vi "BGA244_Main.vi"(7 "stop_external":refnum<vi>, 8 "cluster_ref_BGA244":T1) -> ()   [LabVIEW 2019]
uses:
  cluster_ref_BGA244.ctl
panel:
  in  "Logging":bool=TRUE
  in  "meas_interval":i32=1000 caption="Measurement interval (ms)"
  out "mode":string
  in  "He/Air Mode Button":bool
  out "Purity Meter":dbl(knob) caption="Purity (%)" scale=0.0..100.0 scale format="%#.2f"
  in  "He Mode Button":bool
  in  "O2/N2 Mode Button":bool
  out "gas 2":string
  out "gas 1":string
  out "Purity Chart":waveform(dbl)[](graph)
  out "Status":bool
  in  "VISA":refnum<visa-resource-name>="COM18"
  out "Last measured":timestamp format="%<%Y-%m-%d %H:%M:%S>T"
  in  "Stop":bool
  # "Gas Analyzer Panel"
  # "1333-74-0: H2\n7440-59-7: He\n7727-37-9: N2\n7782-44-7: O2\n7740-37-1: Ar\n132259-10-0: Air"
  # "BGA244"
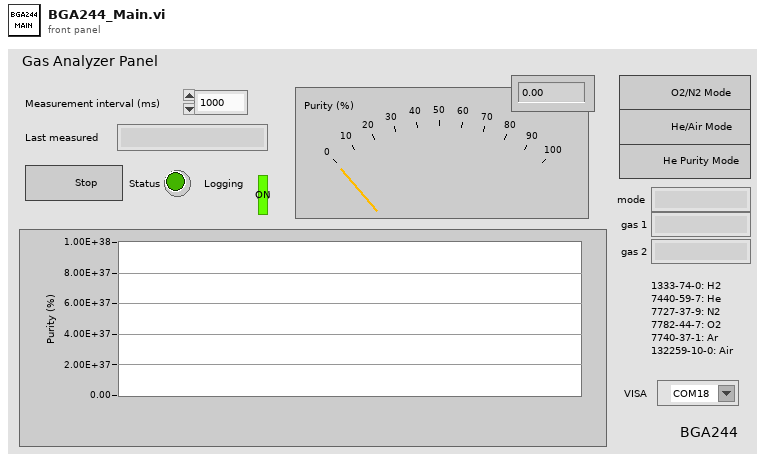
[diagram p1: front panel]
types:
  T1 = typedef "cluster_ref_BGA244.ctl" = cluster{"Status":refnum<vi>, "purity":refnum<vi>}
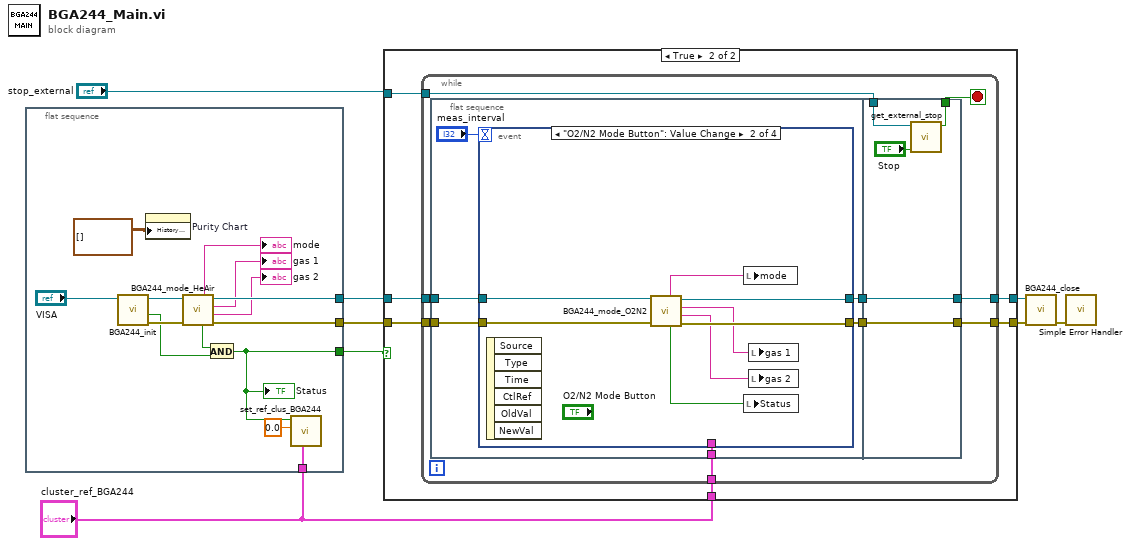
[diagram p0: block diagram]
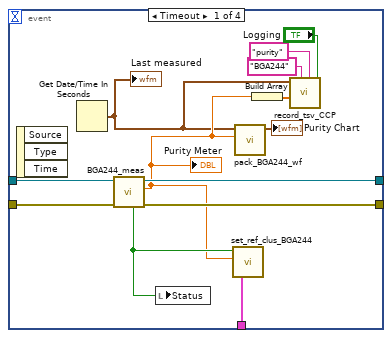
[diagram p3: hidden frame]
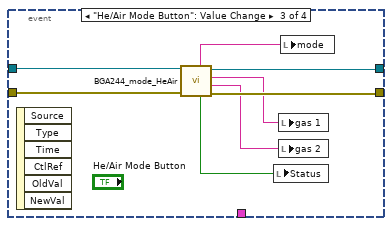
[diagram p4: hidden frame]
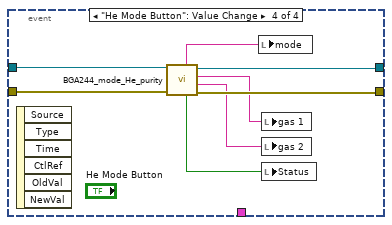
[diagram p5: hidden frame]
diagram:
  n1 = flat-sequence {
    tunnel: [w17] -> w6
    tunnel: [w19] -> w7
    tunnel: "cluster_ref_BGA244" -> [w12]
    tunnel: [w9] -> w1
    frame #0 {
      n2 = call "BGA244_init.vi"("VISA in"="VISA") -> ("error out"=w18:errorcluster, "status"=w14:bool, "VISA out"=w20:refnum<visa-resource-name>)  [unwired: 8 in]
      n3 = property on="Purity Chart" class="WFChart (strict)"("History Data"=waveform(dbl)[][] []) -> ()  [unwired: 2 in, 2 out]
      n4 = call "BGA244_mode_HeAir.vi"("error in"=w18, "VISA in"=w20) -> ("error out"=w17:errorcluster, "gas 2"=→"gas 2":string, "gas 1"=→"gas 1":string, "VISA out"=w19:refnum<visa-resource-name>, "status"=w13:bool, "mode"=→"mode":string)  [unwired: 4 in]
      n5 = And(x=w13, y=w14) -> (x .and. y?=w9:bool)
      "Status" <- w9
      n6 = call "set_ref_clus_BGA244.vi"("cluster_ref_BGA244"=w12, "purity"=0.0, "status"=w9) -> ()  [unwired: 9 in]
    }
  }
  n7 = case shown="True" w1 {
    tunnel: "stop_external" -> [_ w30]
    tunnel: w7 -> [w24 w29]
    tunnel: w6 -> [w23 w28]
    tunnel: [w23 w27] -> w5
    tunnel: [w24 w26] -> w4
    tunnel: "cluster_ref_BGA244" -> [_ w25]
    frame False {
    }
    frame True {
      n8 = while {
        tunnel: w25 -> [w39]
        tunnel: w30 -> [w32]
        tunnel: w29 -> [w38]
        tunnel: w28 -> [w37]
        tunnel: [w36] -> w27
        tunnel: [w35] -> w26
        stop <- w31 stop-if-true
        n9 = flat-sequence {
          tunnel: w39 -> [w45]
          tunnel: w38 -> [w44]
          tunnel: w37 -> [w43]
          tunnel: [w42] -> w34
          tunnel: [w41] -> w33
          tunnel: [w86] -> w35
          tunnel: [w87] -> w36
          tunnel: w34 -> [w87]
          tunnel: w33 -> [w86]
          tunnel: w32 -> [w85]
          tunnel: [w84] -> w31
          frame #0 {
            n10 = event shown="[1] \"O2/N2 Mode Button\": Value Change" {
              selector: _ -> [_ _ _ _]
              dyn-events: _ -> [_ _ _ _]
              timeout: "meas_interval" -> [_ _ _ _]
              tunnel: w45 -> [w58 _ _ _]
              tunnel: w43 -> [w57 w65 w73 w81]
              tunnel: w44 -> [w56 w66 w74 w82]
              tunnel: [w54 w64 w72 w80] -> w41
              tunnel: [w53 w63 w71 w79] -> w42
              event Timeout {
                n11 = event-data() -> ()  [unwired: 1 in, 3 out]
                n12 = Get Date/Time In Seconds() -> (seconds since 1Jan1904=w49:timestamp)
                "Last measured" <- w49
                n13 = call "BGA244_meas.vi"("error in"=w57, "VISA in"=w56) -> ("error out"=w53:errorcluster, "ratio1"=w50:dbl, "VISA out"=w54:refnum<visa-resource-name>, "status"=w52:bool)  [unwired: 5 in, 1 out]
                "Purity Meter" <- w50
                n14 = local write "Status"(w52) -> ()
                n15 = call "set_ref_clus_BGA244.vi"("cluster_ref_BGA244"=w58, "purity"=w50, "status"=w52) -> ()  [unwired: 9 in]
                n16 = call "pack_BGA244_wf.vi"("purity"=w50, "time"=w49) -> ("waveform_array"=→"Purity Chart":waveform(dbl)[])  [unwired: 9 in]
                n17 = Build Array(w50) -> (w51:dbl[])
                n18 = call "record_tsv_CCP.vi"("logging_on"="Logging", "file_name"="purity", "folder_name"="BGA244", "value_array"=w51, "time"=w49) -> ()  [unwired: 5 in, 2 out]
              }
              event "O2/N2 Mode Button": Value Change {
                n19 = event-data() -> ()  [unwired: 1 in, 6 out]
                n20 = call "BGA244_mode_O2N2.vi"("error in"=w65, "VISA in"=w66) -> ("error out"=w63:errorcluster, "gas 2"=w61:string, "gas 1"=w62:string, "VISA out"=w64:refnum<visa-resource-name>, "status"=w60:bool, "mode"=w59:string)  [unwired: 4 in]
                n21 = local write "mode"(w59) -> ()
                n22 = local write "Status"(w60) -> ()
                n23 = local write "gas 1"(w62) -> ()
                n24 = local write "gas 2"(w61) -> ()
              }
              event "He/Air Mode Button": Value Change {
                n25 = event-data() -> ()  [unwired: 1 in, 6 out]
                n26 = call "BGA244_mode_HeAir.vi"("error in"=w73, "VISA in"=w74) -> ("error out"=w71:errorcluster, "gas 2"=w69:string, "gas 1"=w70:string, "VISA out"=w72:refnum<visa-resource-name>, "status"=w68:bool, "mode"=w67:string)  [unwired: 4 in]
                n27 = local write "Status"(w68) -> ()
                n28 = local write "gas 1"(w70) -> ()
                n29 = local write "gas 2"(w69) -> ()
                n30 = local write "mode"(w67) -> ()
              }
              event "He Mode Button": Value Change {
                n31 = event-data() -> ()  [unwired: 1 in, 6 out]
                n32 = call "BGA244_mode_He_purity.vi"("error in"=w81, "VISA in"=w82) -> ("error out"=w79:errorcluster, "gas 2"=w77:string, "gas 1"=w78:string, "VISA out"=w80:refnum<visa-resource-name>, "status"=w76:bool, "mode"=w75:string)  [unwired: 4 in]
                n33 = local write "mode"(w75) -> ()
                n34 = local write "gas 1"(w78) -> ()
                n35 = local write "gas 2"(w77) -> ()
                n36 = local write "Status"(w76) -> ()
              }
            }
          }
          frame #1 {
            n37 = call "get_external_stop.vi"("stop_internal"="Stop", "ref_stop_external"=w85) -> ("stop_output"=w84:bool)  [unwired: 9 in]
          }
        }
      }
    }
  }
  n38 = call "BGA244_close.vi"("error in"=w5, "VISA in"=w4) -> ("error out"=w3:errorcluster)  [unwired: 9 in]
  n39 = call <vilib>:"Simple Error Handler.vi"("error in (no error)"=w3) -> ()  [unwired: 4 in, 5 out]
